vi "FILE_DIALOG.vi"(0 "flow_slope_IN":dbl=51.35 format="%.2f", 1 "pressure_slope_IN":dbl=23.33 format="%.2f", 3 "string_pot_slope_IN":dbl=1.5 format="%.2f", 4 "Descriptions":string[](array[string]), 5 "error in (no error)":errorcluster, 6 "start path":path=path "C:/", 7 "Sensor Cluster":T1, 10 "Array in":refnum<k24>[](array[refnum])) -> (8 "path":path, 9 "Sensor Cluster 2":T1, 11 "exists":bool, 12 "Array out":refnum<k24>[](array[refnum]), 14 "flow_slope_OUT":dbl=51.35 format="%.2f", 15 "pressure_slope_OUT":dbl=732.5347533511234 format="%.2f", 17 "string_pot_slope_OUT":dbl=1.5 format="%.2f", 19 "error out":errorcluster)   [LabVIEW 2016]
uses:
  C:/Program Files (x86)/National Instruments/LabVIEW 2016/vi.lib/ULx/ULx_LV.dll
  Waterloo DAQ/controls/MCC DAQ Readings.ctl
panel:
  out "cal_completed":bool
  out "new_or _prev_file_selected":bool
  in  "calibrate_KPRO":bool
  in  "previous_file":bool
  in  "new_file":bool
  in  "OK Button":bool
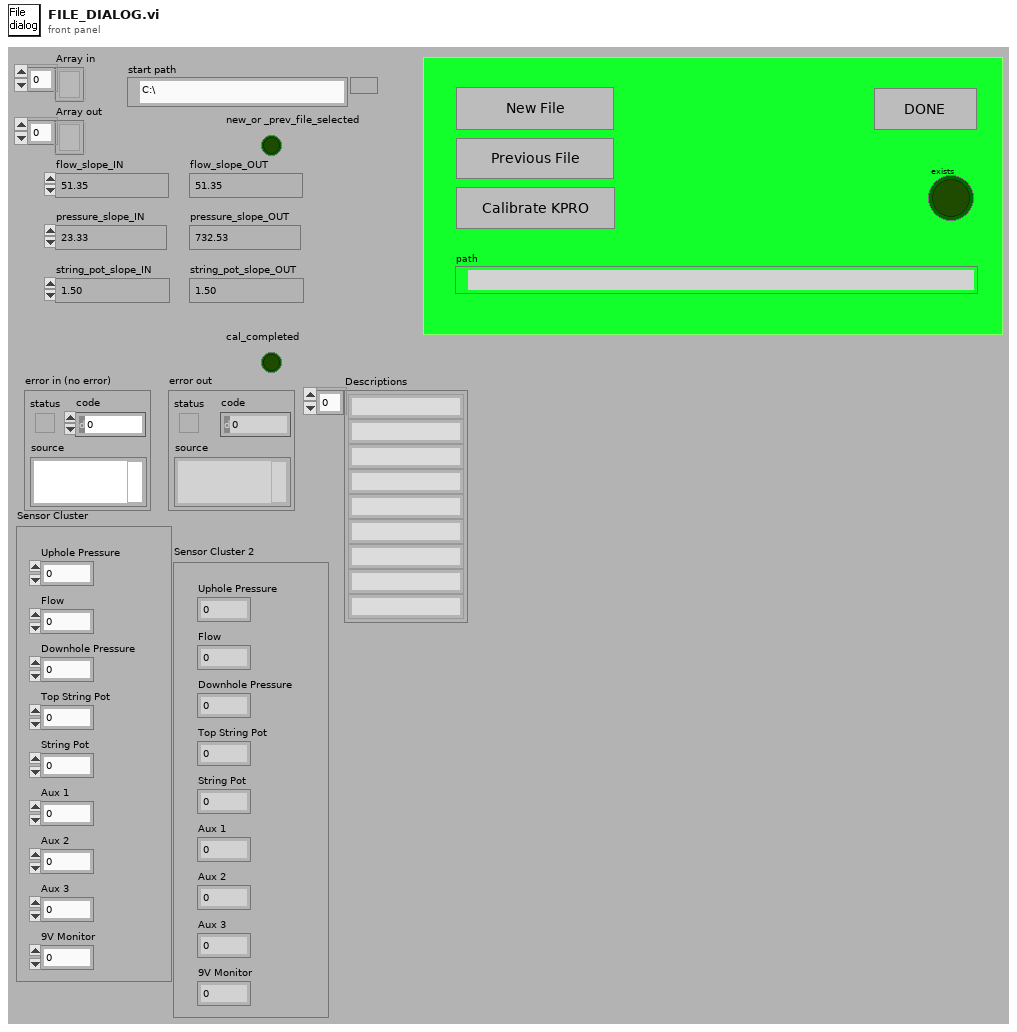
[diagram p1: front panel]
types:
  T1 = typedef "MCC DAQ Readings.ctl" = cluster{"Uphole Pressure":dbl, "Flow":dbl, "Downhole Pressure":dbl, "Top String Pot":dbl, "String Pot":dbl, "Aux 1":dbl, "Aux 2":dbl, "Aux 3":dbl, "9V Monitor":dbl}
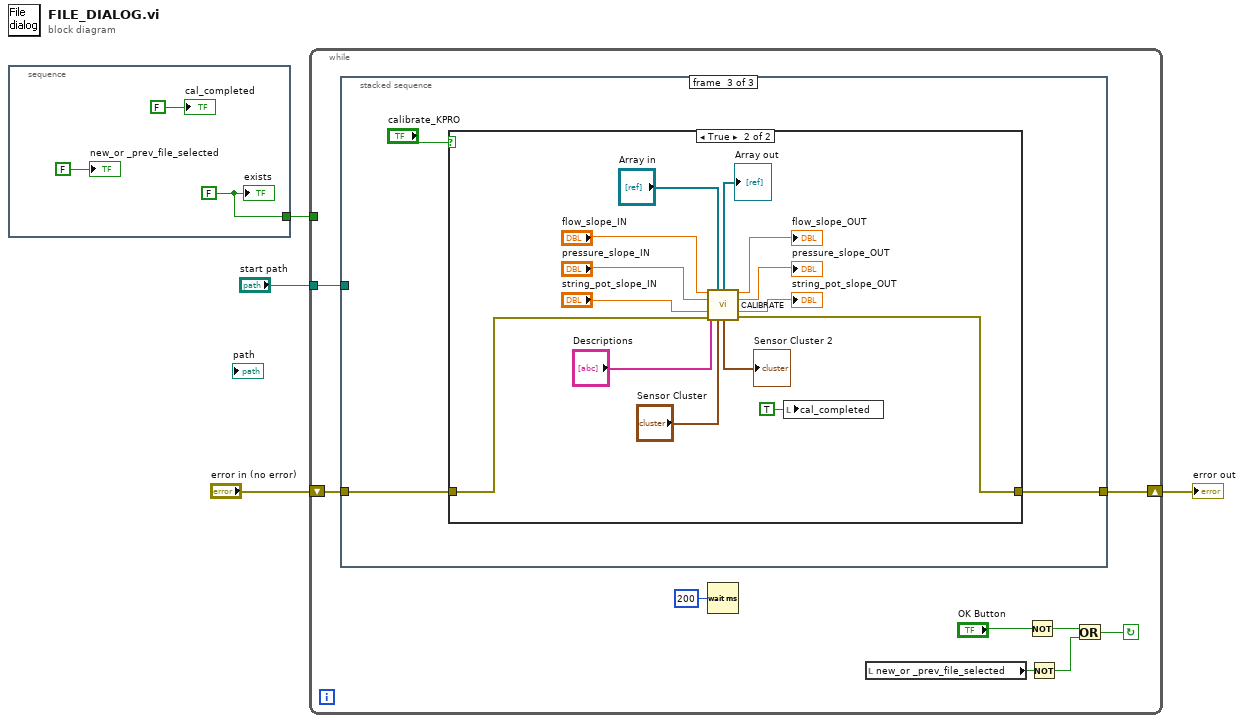
[diagram p0: block diagram]
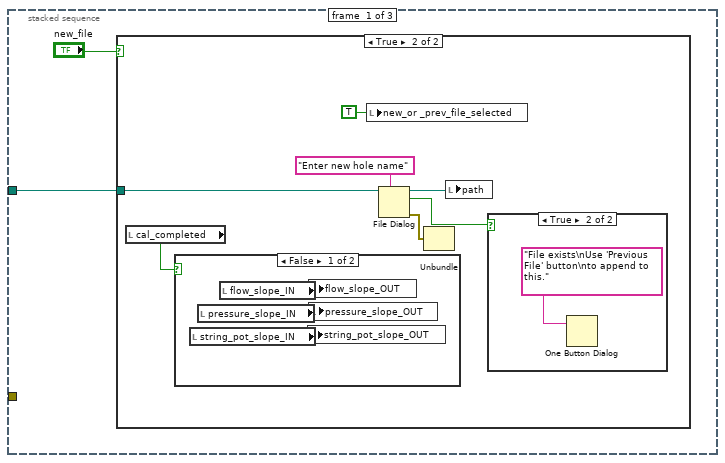
[diagram p2: hidden frame]
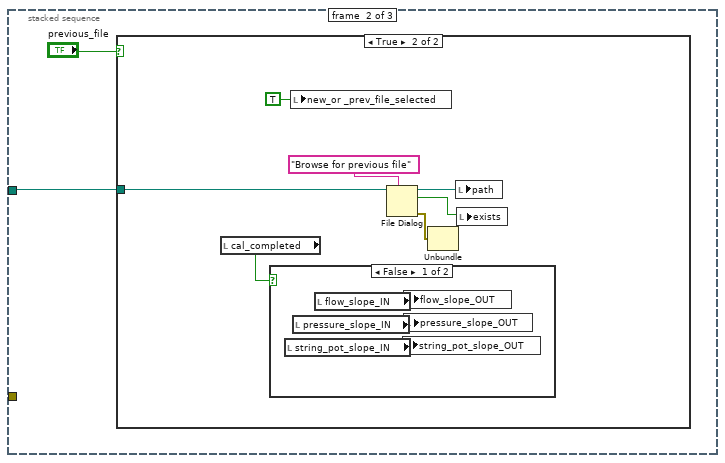
[diagram p6: hidden frame]
diagram:
  n1 = stacked-sequence {
    tunnel: [w7] -> w4
    frame #0 {
      w7 = FALSE ("exists")
      "exists" <- w7
      "new_or _prev_file_selected" <- FALSE ("new_or _prev_file_selected")
      "cal_completed" <- FALSE ("cal_completed")
    }
  }
  n2 = while {
    shift-left: "error in (no error)" -> [w13]
    shift-right: [w12] -> w1
    tunnel: "start path" -> [w14]
    tunnel: w4 -> [_]
    stop <- w11 continue-if-true
    n3 = stacked-sequence {
      tunnel: w14 -> [w17 w30 _]
      tunnel: w13 -> [_ _ w43]
      tunnel: [_ _ w42] -> w12
      frame #0 {
        n4 = case shown="True" "new_file" {
          tunnel: w17 -> [_ w22]
          frame False {
          }
          frame True {
            n5 = local read "cal_completed"() -> (w20:bool)
            n6 = case shown="False" w20 {
              frame False {
                n7 = local read "string_pot_slope_IN"() -> (w26:dbl)
                n8 = local read "pressure_slope_IN"() -> (w27:dbl)
                n9 = local read "flow_slope_IN"() -> (w28:dbl)
                n10 = local write "string_pot_slope_OUT"(w26) -> ()
                n11 = local write "flow_slope_OUT"(w28) -> ()
                n12 = local write "pressure_slope_OUT"(w27) -> ()
              }
              frame True {
              }
            }
            n13 = local write "new_or _prev_file_selected"(TRUE ("new_or _prev_file_selected")) -> ()
            n14 = File Dialog(7:"Enter new hole name" ("prompt"), 11:w22) -> (0:w19:errorcluster, 2:w23:bool, 3:w24:path)  [unwired: 5 in, 1 out]
            n15 = Unbundle(w19) -> ()  [unwired: 3 out]
            n16 = local write "path"(w24) -> ()
            n17 = case shown="True" w23 {
              frame False {
              }
              frame True {
                n18 = One Button Dialog(message="File exists\nUse 'Previous File' button\nto append to this.") -> ()  [unwired: 1 in, 1 out]
              }
            }
          }
        }
      }
      frame #1 {
        n19 = case shown="True" "previous_file" {
          tunnel: w30 -> [_ w35]
          frame False {
          }
          frame True {
            n20 = local read "cal_completed"() -> (w33:bool)
            n21 = case shown="False" w33 {
              frame False {
                n22 = local read "string_pot_slope_IN"() -> (w39:dbl)
                n23 = local read "pressure_slope_IN"() -> (w40:dbl)
                n24 = local read "flow_slope_IN"() -> (w41:dbl)
                n25 = local write "string_pot_slope_OUT"(w39) -> ()
                n26 = local write "flow_slope_OUT"(w41) -> ()
                n27 = local write "pressure_slope_OUT"(w40) -> ()
              }
              frame True {
              }
            }
            n28 = local write "new_or _prev_file_selected"(TRUE ("new_or _prev_file_selected")) -> ()
            n29 = File Dialog(7:"Browse for previous file" ("prompt"), 11:w35) -> (0:w32:errorcluster, 2:w36:bool, 3:w37:path)  [unwired: 5 in, 1 out]
            n30 = Unbundle(w32) -> ()  [unwired: 3 out]
            n31 = local write "path"(w37) -> ()
            n32 = local write "exists"(w36) -> ()
          }
        }
      }
      frame #2 {
        n33 = case shown="True" "calibrate_KPRO" {
          tunnel: w43 -> [w45 w56]
          tunnel: [w45 w55] -> w42
          frame False {
          }
          frame True {
            n34 = call "CALIBRATE.vi"("flow_slope_IN"="flow_slope_IN", "Array in"="Array in", "pressure_slope_IN"="pressure_slope_IN", "Descriptions"="Descriptions", "string_pot_slope_IN"="string_pot_slope_IN", "error in (no error)"=w56, "Sensor Cluster"="Sensor Cluster") -> ("Array out"=→"Array out":refnum<k24>[], "flow_slope_OUT"=→"flow_slope_OUT":dbl, "pressure_slope_OUT"=→"pressure_slope_OUT":dbl, "string_pot_slope_OUT"=→"string_pot_slope_OUT":dbl, "Sensor Cluster 2"=→"Sensor Cluster 2":T1, "error out"=w55:errorcluster)  [unwired: 3 in]
            n35 = local write "cal_completed"(TRUE ("cal_completed")) -> ()
          }
        }
      }
    }
    n36 = Wait (ms)(milliseconds to wait=u32 200) -> ()  [unwired: 1 out]
    n37 = local read "new_or _prev_file_selected"() -> (w9:bool)
    n38 = Not(x="OK Button") -> (.not. x?=w10:bool)
    n39 = Not(x=w9) -> (.not. x?=w8:bool)
    n40 = Or(x=w10, y=w8) -> (x .or. y?=w11:bool)
  }
  "error out" <- w1
